vi "cDAQ Panel Color Set Ver2.vi"(3 "TC Min OK Val":dbl, 4 "TC Max OK Val":dbl, 5 "StDev Thresh":dbl, 6 "Input Block":T1[](array[typedef])) -> (2 "Output Block":T1[](array[typedef]))   [LabVIEW 2014]
doc: "Check if measurement's mean and std dev are within the defined limits"
uses:
  Type Definitions/cDAQ Instrument Sensor.ctl
panel:
  out "Output Test":T1
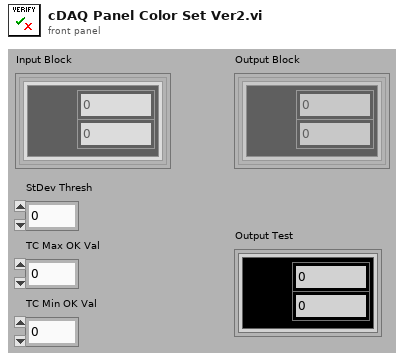
[diagram p1: front panel]
types:
  T1 = typedef "cDAQ Instrument Sensor.ctl" = cluster{"Mean":dbl, " Std":dbl, "Color Box":u32}
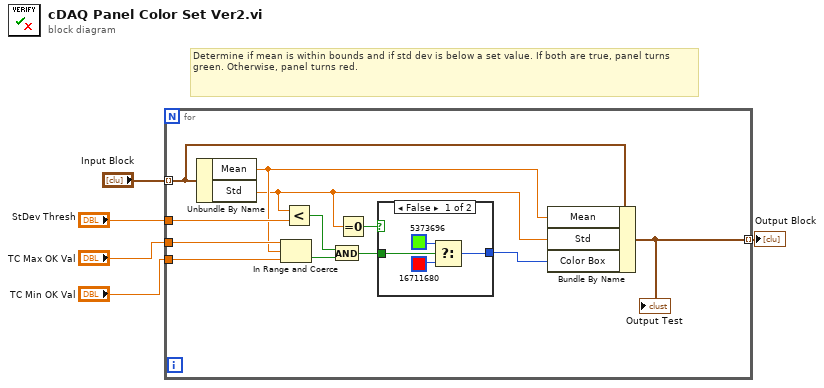
[diagram p0: block diagram]
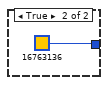
[diagram p2: hidden frame]
diagram:
  # "Determine if mean is within bounds and if std dev is below a set value. If both are true, panel turns green. Otherwise, panel turns red."
  n1 = for {
    tunnel: [w17] -> w1 mode=indexing
    tunnel: "Input Block" -> [w16] mode=indexing
    tunnel: "TC Max OK Val" -> [w15]
    tunnel: "TC Min OK Val" -> [w14]
    tunnel: "StDev Thresh" -> [w13]
    n2 = Unbundle By Name(w16) -> ("Mean"=w10:dbl, "Std"=w7:dbl)
    n3 = In Range and Coerce(upper limit=w15, x=w10, lower limit=w14) -> (In Range?=w9:bool)  [unwired: 1 out]
    n4 = Less?(x=w7, y=w13) -> (x < y?=w12:bool)
    n5 = And(x=w12, y=w9) -> (x .and. y?=w11:bool)
    n6 = Equal To 0?(x=w7) -> (x = 0?=w6:bool)
    n7 = case shown="False" w6 {
      tunnel: [w19 u32 16763136 ("Color Box")] -> w8
      tunnel: w11 -> [w18 _]
      frame False {
        n8 = Select(t=u32 5373696 ("Color Box"), s=w18, f=u32 16711680 ("Color Box")) -> (s? t:f=w19:u32)
      }
      frame True {
      }
    }
    n9 = Bundle By Name(cluster=w16, "Mean"=w10, "Std"=w7, "Color Box"=w8) -> (w17:T1)
    "Output Test" <- w17
  }
  "Output Block" <- w1
